vi "YAML to Tree.vi"(4 "Condensed?":bool=TRUE, 6 "VI Refnum":refnum<vi>, 8 "error in (no error)":errorcluster, 10 "Tree Refnum":refnum<vi>, 11 "YAML Parser in":refnum<class "YAML Parser.lvclass">) -> (0 "error out":errorcluster, 3 "YAML Parser out":refnum<class "YAML Parser.lvclass">)   [LabVIEW 2015, in "YAML Parser.lvclass"]
uses:
  YAML Parser.lvclass
  YAML Parser.lvclass/YAML Parser.ctl
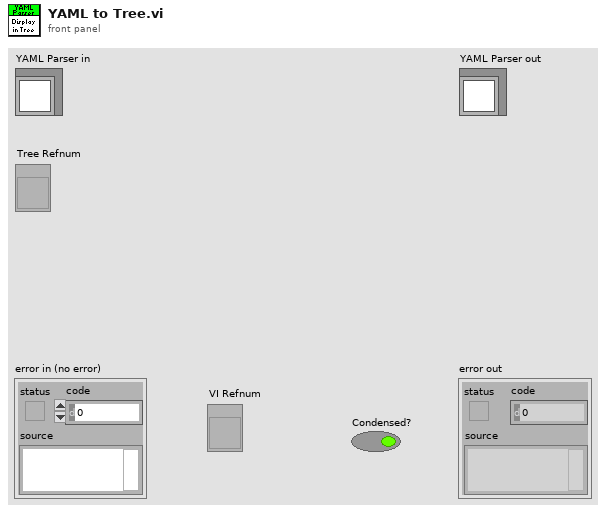
[diagram p1: front panel]
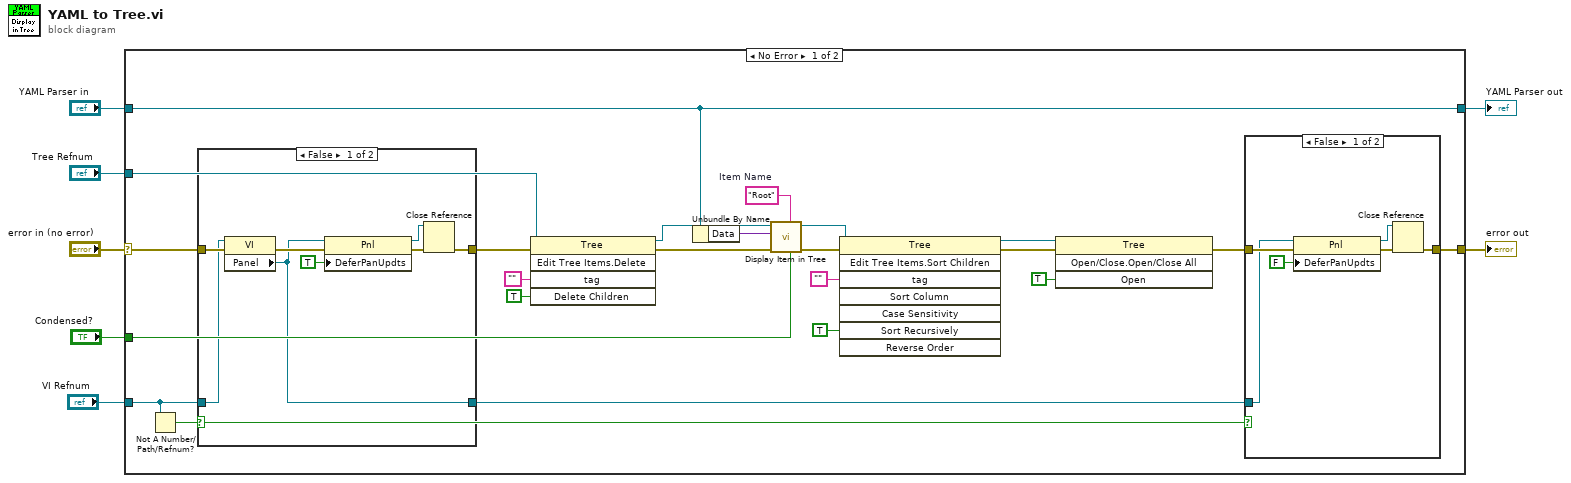
[diagram p0: block diagram]
diagram:
  n1 = case shown="No Error" "error in (no error)" {
    selector: "error in (no error)" -> [w14 w48]
    tunnel: [w9 w48] -> w6
    tunnel: [w27 w47] -> w4
    tunnel: "YAML Parser in" -> [w27 w47]
    tunnel: "Tree Refnum" -> [w30 _]
    tunnel: "Condensed?" -> [w15 _]
    tunnel: "VI Refnum" -> [w12 _]
    frame No Error {
      w18 = "Root"  # Item Name
      n2 = Not A Number/Path/Refnum?(number/path/refnum=w12) -> (NaN/Path/Refnum?=w11:bool)
      n3 = case shown="False" w11 {
        tunnel: w14 -> [w43 w46]
        tunnel: [w42 w46] -> w13
        tunnel: w12 -> [w39 _]
        tunnel: [w38 _] -> w8
        frame False {
          n4 = property class="VI"(reference=w39, error in=w43) -> (error out=w40:errorcluster, "Panel"=w38:refnum<vi>)  [unwired: 1 out]
          n5 = property class="Pnl"(reference=w38, error in=w40, "DeferPanUpdts"=TRUE ("Defer Panel Updates")) -> (reference out=w45:refnum<vi>, error out=w44:errorcluster)
          n6 = Close Reference(reference=w45, error in (no error)=w44) -> (error out=w42:errorcluster)
        }
        frame True {
        }
      }
      n7 = invoke class="Tree" method="Edit Tree Items.Delete"(reference=w30, error in=w13, "tag"="", "Delete Children"=TRUE) -> (reference out=w24:refnum<vi>, error out=w26:errorcluster)  [unwired: 1 in, 3 out]
      n8 = Unbundle By Name(w27) -> ("Data"=w25:variant)
      n9 = call "Display Item in Tree.vi"("Condensed?"=w15, "Item Name"=w18, "error in (no error)"=w26, "Data"=w25, "Tree Refnum"=w24) -> ("error out"=w23:errorcluster, "Tree Refnum out"=w20:refnum<vi>)  [unwired: 5 in]
      n10 = invoke class="Tree" method="Edit Tree Items.Sort Children"(reference=w20, error in=w23, "tag"="", "Sort Recursively"=TRUE) -> (reference out=w22:refnum<vi>, error out=w21:errorcluster)  [unwired: 4 in, 6 out]
      n11 = invoke class="Tree" method="Open/Close.Open/Close All"(reference=w22, error in=w21, "Open"=TRUE) -> (error out=w10:errorcluster)  [unwired: 1 in, 3 out]
      n12 = case shown="False" w11 {
        tunnel: w10 -> [w34 w37]
        tunnel: [w33 w37] -> w9
        tunnel: w8 -> [w32 _]
        frame False {
          n13 = property class="Pnl"(reference=w32, error in=w34, "DeferPanUpdts"=FALSE ("Defer Panel Updates")) -> (reference out=w35:refnum<vi>, error out=w36:errorcluster)
          n14 = Close Reference(reference=w35, error in (no error)=w36) -> (error out=w33:errorcluster)
        }
        frame True {
        }
      }
    }
    frame Error {
    }
  }
  "error out" <- w6
  "YAML Parser out" <- w4
